vi "Search string for key string by bytes.vi"(8 "error in (no error)":errorcluster, 9 "offset":u32, 10 "Search for string":string, 11 "String":string) -> (0 "error out":errorcluster, 1 "Offset past match":i32, 2 "After":string, 3 "Before":string, 5 "Found match?":bool)   [LabVIEW 2024]
panel:
  out "offset of match":i32
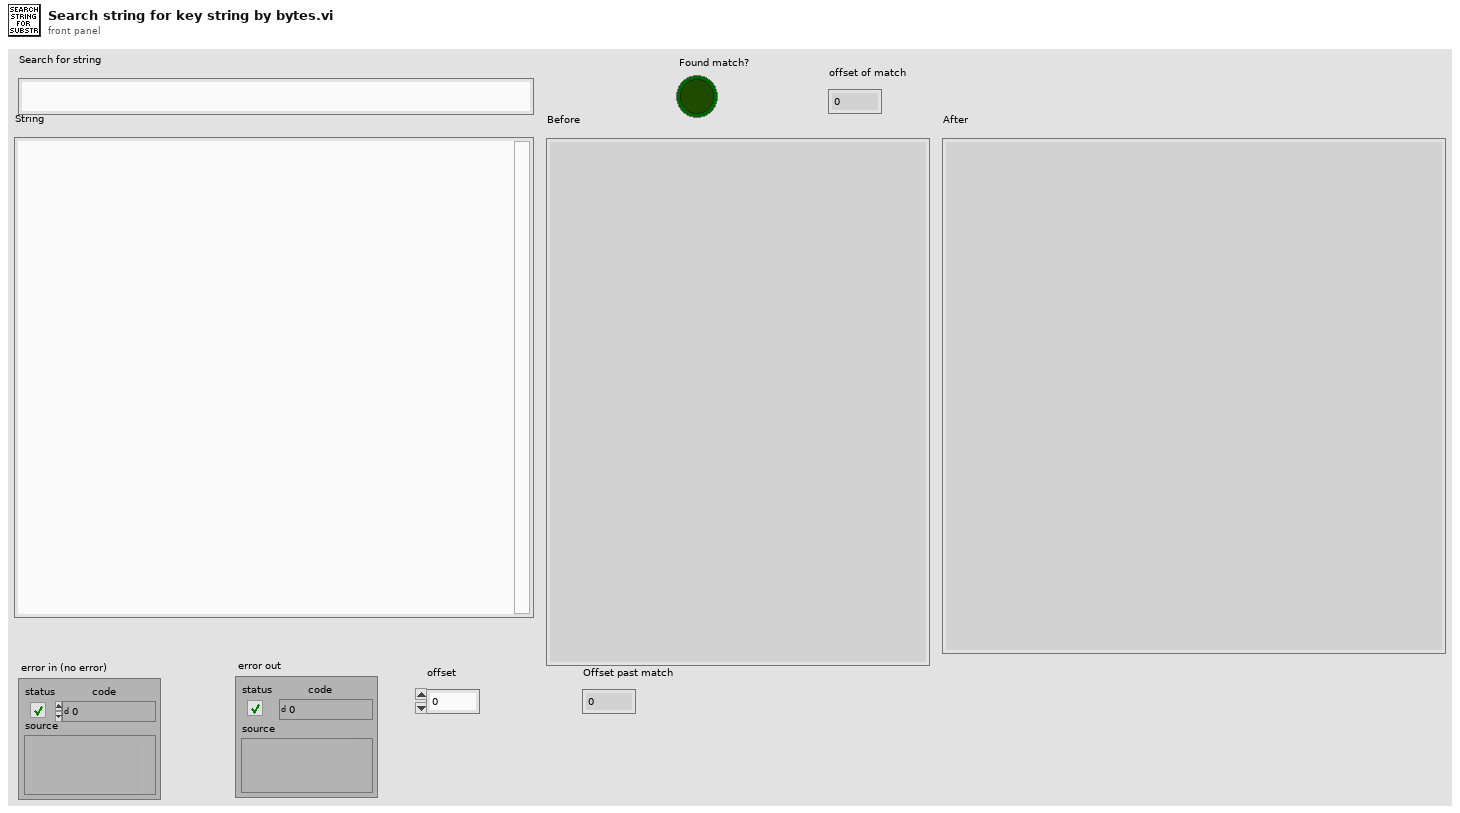
[diagram p1: front panel]
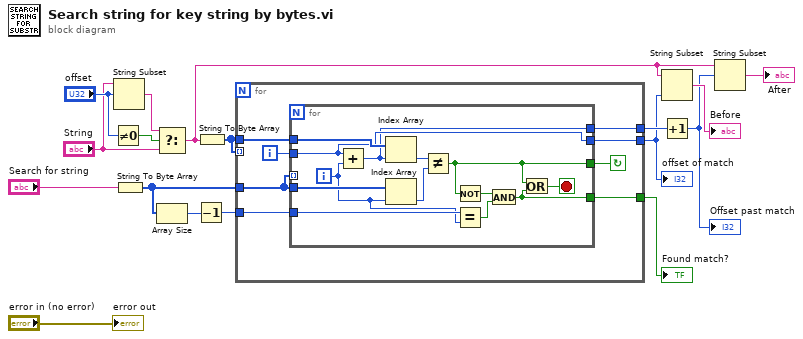
[diagram p0: block diagram]
diagram:
  n1 = Not Equal To 0?(x="offset") -> (x != 0?=w6:bool)
  n2 = String Subset(string="String", offset (0)="offset") -> (substring=w4:string)  [unwired: 1 in]
  n3 = String To Byte Array(string="Search for string") -> (unsigned byte array=w15:u8[])
  n4 = Select(t=w4, s=w6, f="String") -> (s? t:f=w1:string)
  n5 = Array Size(array=w15) -> (size(s)=w14:i32)
  n6 = Decrement(x=w14) -> (x-1=w13:i32)
  n7 = String To Byte Array(string=w1) -> (unsigned byte array=w17:u8[])
  n8 = for {
    tunnel: w17 -> [_] mode=indexing
    tunnel: w15 -> [w23]
    tunnel: w17 -> [w25]
    tunnel: [w18] -> w16
    tunnel: [w21] -> w12
    tunnel: w13 -> [w20]
    tunnel: [w19] -> w10
    i -> [w24]
    stop <- w22 continue-if-true
    n9 = for {
      tunnel: w23 -> [_] mode=indexing
      tunnel: w25 -> [w38]
      tunnel: w24 -> [w30]
      tunnel: w23 -> [w37]
      tunnel: [w28] -> w22
      tunnel: [w26] -> w21
      tunnel: w20 -> [w35]
      tunnel: [w30] -> w19
      tunnel: [w27] -> w18
      i -> [w34]
      stop <- w31 stop-if-true
      n10 = Add(x=w30, y=w34) -> (x+y=w26:i32)
      n11 = Index Array(array=w38, index=w26) -> (element=w29:u8)
      n12 = Index Array(array=w37, index=w34) -> (element=w36:u8)
      n13 = Not Equal?(x=w29, y=w36) -> (x != y?=w28:bool)
      n14 = Not(x=w28) -> (.not. x?=w33:bool)
      n15 = Equal?(x=w35, y=w34) -> (x = y?=w32:bool)
      n16 = And(x=w33, y=w32) -> (x .and. y?=w27:bool)
      n17 = Or(x=w28, y=w27) -> (x .or. y?=w31:bool)
    }
  }
  "Found match?" <- w16
  "offset of match" <- w10
  n18 = String Subset(string=w1, length (rest)=w10) -> (substring=→"Before":string)  [unwired: 1 in]
  n19 = Increment(x=w12) -> (x+1=w8:i32)
  "Offset past match" <- w8
  n20 = String Subset(string=w1, offset (0)=w8) -> (substring=→"After":string)  [unwired: 1 in]
  "error out" <- "error in (no error)"
